vi "Create Channels.vi"(7 "I/O Type":enum16{"Voltage AO", "Voltage AI"}(ring), 8 "error in (no error)":errorcluster, 9 "Stimulus Outputs":T1, 10 "Instrument Specifications":T8, 11 "Refnum in":refnum<k21>) -> (0 "error out":errorcluster, 3 "Refnum out":refnum<k21>)   [LabVIEW 2026, in "Acquisition.lvlib"]
uses:
  Acquisition.lvlib
  Instrument Specifications Configuration.ctl
  Instrument Specifications Cluster Configuration.ctl
  controls/UI/Measurement Role.ctl
  controls/Controller/Stimulus Outputs.ctl
  controls/Controller/Stimulus Output.ctl
  controls/Controller/Controller Core Data.ctl
  controls/UI/Units Enum.ctl
  controls/UI/Signal Enum.ctl
  controls/Controller/Stimulus Output Configuration.ctl
  controls/Controller/Stimulus Role.ctl
  <vilib>/DAQmx/create/channels.llb/DAQmx Create Channel (AI-Voltage-Basic).vi
  <vilib>/DAQmx/create/channels.llb/DAQmx Create Channel (AO-Voltage-Basic).vi
  Settings/Settings.lvlib
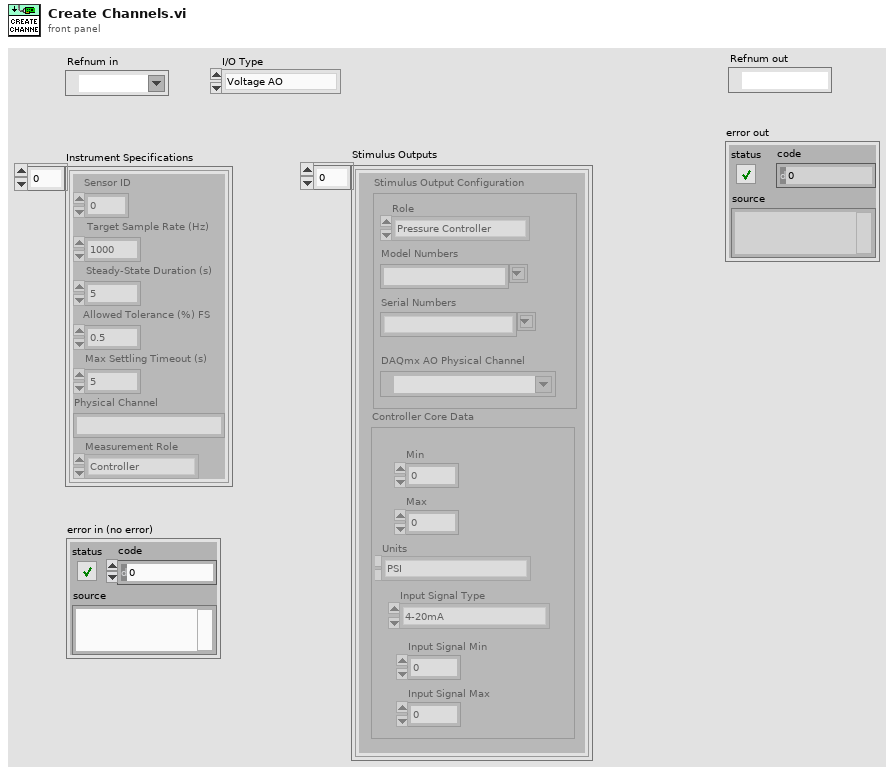
[diagram p1: front panel]
types:
  T1 = typedef "Settings.lvlib/Stimulus Outputs.ctl" = T2[]
  T2 = typedef "Settings.lvlib/Stimulus Output.ctl" = cluster{"Controller Core Data":T3, "Stimulus Output Configuration":T6}
  T3 = typedef "Settings.lvlib/Controller Core Data.ctl" = cluster{"Min":dbl, "Max":dbl, "Units":T4, "Input Signal Type":T5, "Input Signal Min":dbl, "Input Signal Max":dbl}
  T4 = typedef "Units Enum.ctl" = enum16{"PSI", "Deg C", "kPa", "GPM"}
  T5 = typedef "Signal Enum.ctl" = enum16{"4-20mA", "0-10V", "Thermocouple Type K"}
  T6 = typedef "Settings.lvlib/Stimulus Output Configuration.ctl" = cluster{"DAQmx AO Physical Channel":tag, "Role":T7, "Model Numbers":string, "Serial Numbers":string}
  T7 = typedef "Stimulus Role.ctl" = enum16{"Pressure Controller", "Temperature Controller"}
  T8 = typedef "Acquisition.lvlib/Instrument Specifications Configuration.ctl" = T9[]
  T9 = typedef "Acquisition.lvlib/Instrument Specifications Cluster Configuration.ctl" = cluster{"Sensor ID":i32, "Target Sample Rate (Hz)":dbl, "Steady-State Duration (s)":i32, "Allowed Tolerance (%) FS":dbl, "Max Settling Timeout (s)":i32, "Physical Channel":string, "Measurement Role":T10}
  T10 = typedef "Settings.lvlib/Measurement Role.ctl" = enum16{"Controller", "Reference", "UUT", "Disable", "All"}
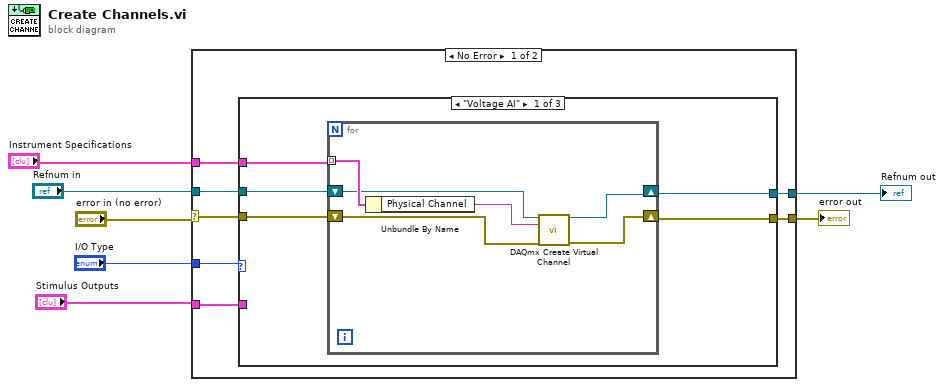
[diagram p0: block diagram]
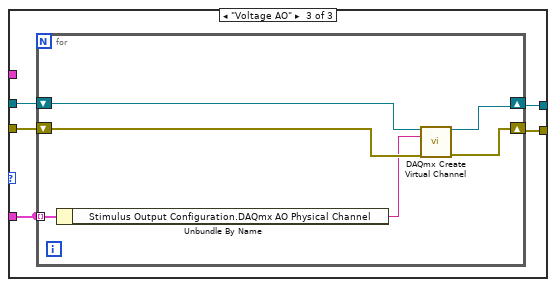
[diagram p3: hidden frame]
diagram:
  n1 = case shown="No Error" "error in (no error)" {
    selector: "error in (no error)" -> [w10 w41]
    tunnel: "Refnum in" -> [w14 w42]
    tunnel: "Instrument Specifications" -> [w13 _]
    tunnel: [w12 w42] -> w5
    tunnel: [w11 w41] -> w4
    tunnel: "I/O Type" -> [w9 _]
    tunnel: "Stimulus Outputs" -> [w8 _]
    frame No Error {
      n2 = case shown="\"Voltage AI\"" w9 {
        tunnel: w14 -> [w20 w28 w34]
        tunnel: w13 -> [w19 _ _]
        tunnel: [w18 w28 w33] -> w12
        tunnel: [w17 w27 w32] -> w11
        tunnel: w10 -> [w16 w27 w31]
        tunnel: [w15 w29 w30] -> _
        tunnel: w8 -> [w15 w29 w30]
        frame "Voltage AI" {
          n3 = for {
            shift-right: [w26] -> w17
            shift-left: w16 -> [w23]
            tunnel: w19 -> [w24] mode=indexing
            shift-right: [w25] -> w18
            shift-left: w20 -> [w21]
            n4 = Unbundle By Name(w24) -> ("Physical Channel"=w22:string)
            n5 = call-poly <vilib>:"DAQmx Create Virtual Channel.vi"("task in"=w21, "physical channels"=w22, "error in"=w23) -> ("task out"=w25:refnum<k21>, "error out"=w26:errorcluster)  [unwired: 11 in]
          }
        }
        frame Default {
        }
        frame "Voltage AO" {
          n6 = for {
            shift-right: [w40] -> w32
            shift-left: w31 -> [w38]
            shift-right: [w39] -> w33
            shift-left: w34 -> [w37]
            tunnel: w30 -> [w36] mode=indexing
            n7 = Unbundle By Name(w36) -> ("Stimulus Output Configuration.DAQmx AO Physical Channel"=w35:tag)
            n8 = call-poly <vilib>:"DAQmx Create Virtual Channel.vi"("task in"=w37, "physical channels"=w35, "error in"=w38) -> ("task out"=w39:refnum<k21>, "error out"=w40:errorcluster)  [unwired: 11 in]
          }
        }
      }
    }
    frame Error {
    }
  }
  "Refnum out" <- w5
  "error out" <- w4
